vi "control de servo.vi"() -> ()   [LabVIEW 2016]
uses:
  <vilib>/LabVIEW Interface for Arduino/Type Defs/Board Type.ctl
  <vilib>/LabVIEW Interface for Arduino/Type Defs/Connection Type.ctl
  <vilib>/LabVIEW Interface for Arduino/LabVIEW Interface for Arduino.lvlib
panel:
  out "Angle (Degrees)":u8=15
  in  "stop":bool
  in  "Dial":u32(knob) scale=0.0..180.0
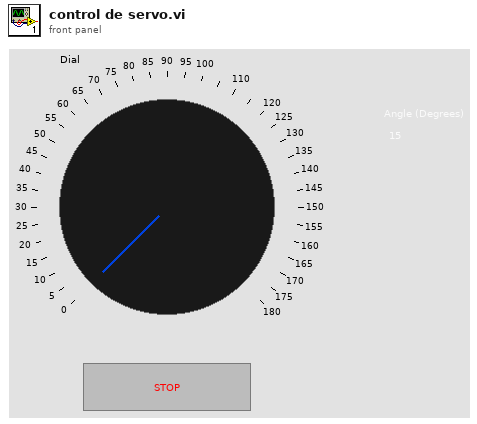
[diagram p1: front panel]
types:
  T1 = typedef "LabVIEW Interface for Arduino.lvlib/Connection Type.ctl" = enum8{"USB / Serial", "XBEE", "BlueSmirf (Bluetooth)"}
  T2 = typedef "LabVIEW Interface for Arduino.lvlib/Board Type.ctl" = enum16{"Uno", "Dimuelanove w/Atmega 328", "Mega 2560"}
  T3 = typedef "LabVIEW Interface for Arduino.lvlib/Arduino Resource.ctl" = cluster{"VISA resource":refnum<visa-resource-name>, "Board Type":T2, "Connection Type":enum8{"USB / Serial"}, "Bytes Per Packet (15)":u8}
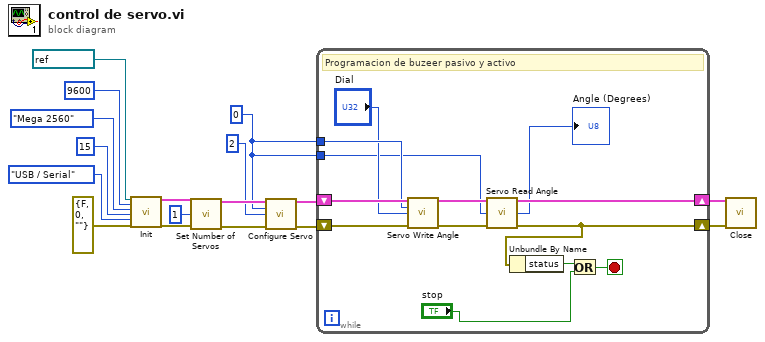
[diagram p0: block diagram]
diagram:
  w1 = u8 0 ("Servo Number (0)")
  n1 = call <vilib>:"Init.vi"("VISA resource"=refnum<visa-resource-name> "COM6", "Baud Rate (115200)"=u32 9600, "Board Type (Uno)"=Board_Type."Mega 2560", "Bytes Per Packet (15)"=u32 15, "Connection Type (USB/Serial)"=Connection_Type."USB / Serial", "error in"=errorcluster {"status"=FALSE, "code"=0, "source"=""}) -> ("Arduino Resource"=w8:T3, "error out"=w9:errorcluster)  [unwired: 12 in]
  n2 = call <vilib>:"Set Number of Servos.vi"("Arduino Resource"=w8, "Number Of Servos (1)"=u8 1, "error in"=w9) -> ("Arduino Resource"=w6:T3, "error out"=w5:errorcluster)  [unwired: 11 in]
  n3 = call <vilib>:"Configure Servo.vi"("Arduino Resource"=w6, "Servo Number (0)"=w1, "DIO Pin (2)"=u8 2, "error in"=w5) -> ("Arduino Resource"=w3:T3, "error out"=w2:errorcluster)  [unwired: 10 in]
  n4 = while {
    shift-right: [w24] -> w10
    shift-left: w3 -> [w27]
    shift-right: [w25] -> w11
    shift-left: w2 -> [w26]
    tunnel: w1 -> [w21]
    tunnel: w1 -> [w19]
    stop <- w29 stop-if-true
    # "Programacion de buzeer pasivo y activo"
    n5 = call <vilib>:"Servo Write Angle.vi"("Arduino Resource"=w27, "Servo Number"=w21, "Angle (Degrees)"="Dial", "error in"=w26) -> ("Arduino Resource"=w23:T3, "error out"=w22:errorcluster)  [unwired: 10 in]
    n6 = call <vilib>:"Servo Read Angle.vi"("Arduino Resource"=w23, "Servo Number"=w19, "error in"=w22) -> ("Arduino Resource"=w24:T3, "Angle (Degrees)"=→"Angle (Degrees)":u8, "error out"=w25:errorcluster)  [unwired: 10 in]
    n7 = Unbundle By Name(w25) -> ("status"=w30:bool)
    n8 = Or(x=w30, y="stop") -> (x .or. y?=w29:bool)
  }
  n9 = call <vilib>:"Close.vi"("Arduino Resource"=w10, "error in"=w11) -> ()  [unwired: 13 in, 1 out]
